vi "Create VI.vi"(8 "error in (no error)":errorcluster, 11 "Application in":refnum<vi>) -> (0 "error out":errorcluster, 2 "New VI":refnum<vi>, 3 "Application out":refnum<vi>)   [LabVIEW 2019, in "VI Scripting Utilities.lvlib"]
uses:
  VI Scripting Utilities.lvlib
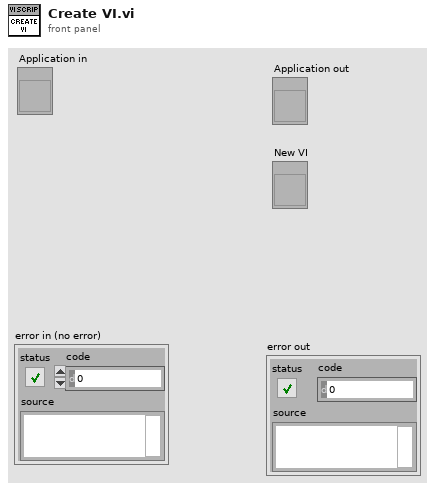
[diagram p1: front panel]
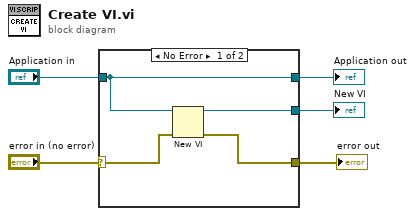
[diagram p0: block diagram]
diagram:
  n1 = case shown="No Error" "error in (no error)" {
    selector: "error in (no error)" -> [w7 w10]
    tunnel: "Application in" -> [w6 w11]
    tunnel: [w9 w10] -> w4
    tunnel: [w8 _] -> w3
    tunnel: [w6 w11] -> w1
    frame No Error {
      n2 = New VI(8:w7, 11:w6) -> (0:w9:errorcluster, 3:w8:refnum<vi>)  [unwired: 5 in]
    }
    frame Error {
    }
  }
  "error out" <- w4
  "New VI" <- w3
  "Application out" <- w1
